vi "System_2.vi"() -> ()   [LabVIEW 2020]
doc: "Use this template to build a producer/consumer design pattern with events to produce queue items. Use this design pattern instead of the User Interface Event Handler pattern for user interfaces when you want to execute code asynchronously in response to an event without slowing the user interface responsiveness."
uses:
  <vilib>/Instr/_visa.llb/VISA Configure Serial Port (Instr).vi
panel:
  out "read data":string
  in  "Low LDR":dbl(slide) scale=0.0..1023.0
  in  "High LDR":dbl(slide) scale=0.0..1023.0
  out "Reward Servo":i32(knob) scale=0.0..180.0
  out "Forward Servo":i32(knob) scale=0.0..180.0
  in  "Baud rate (9600)":u32=9600
  in  "VISA resource name":refnum<visa-resource-name>
  in  "Close":bool
  in  "Open":bool
  out "Connected":bool
  in  "stop":bool
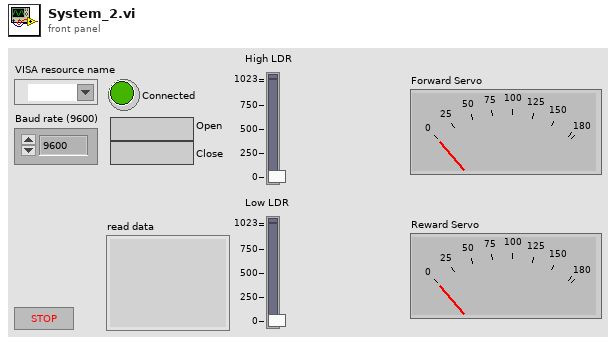
[diagram p1: front panel]
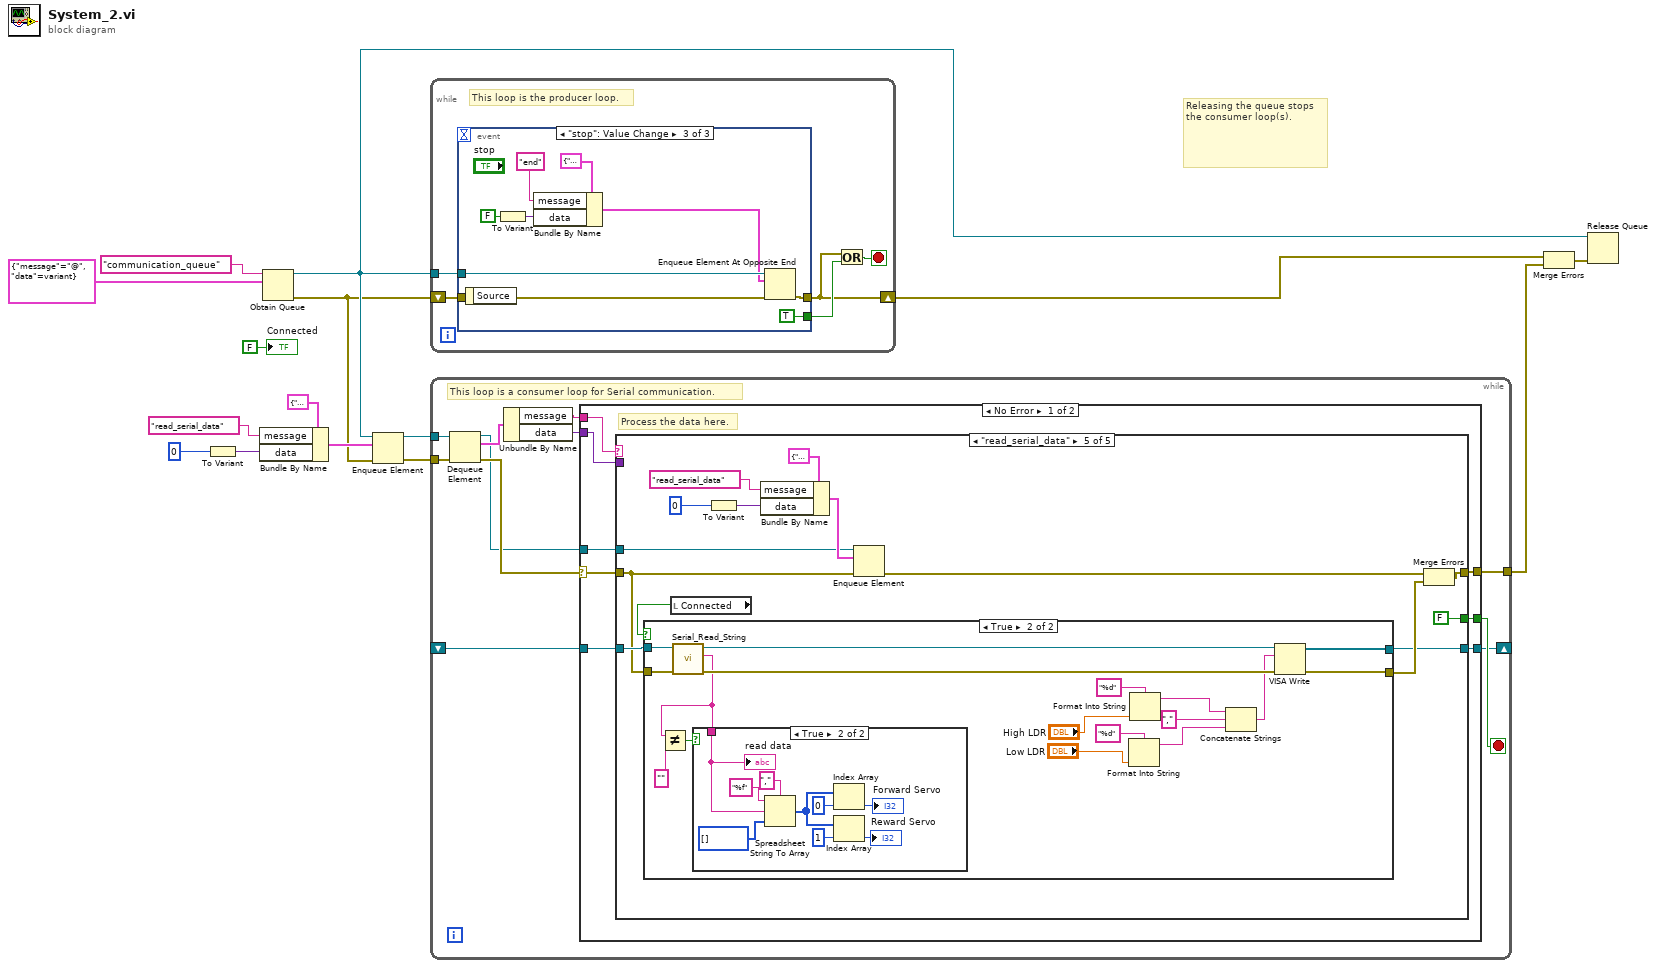
[diagram p0: block diagram]
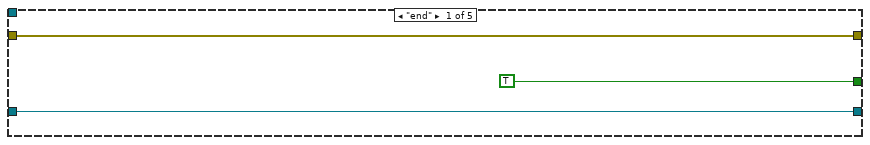
[diagram p2: hidden frame]
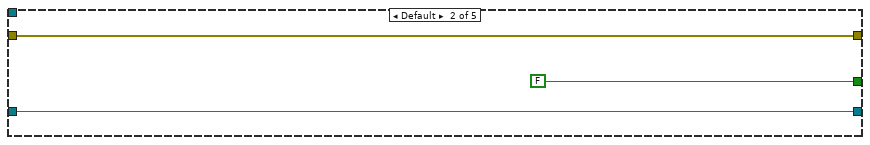
[diagram p3: hidden frame]
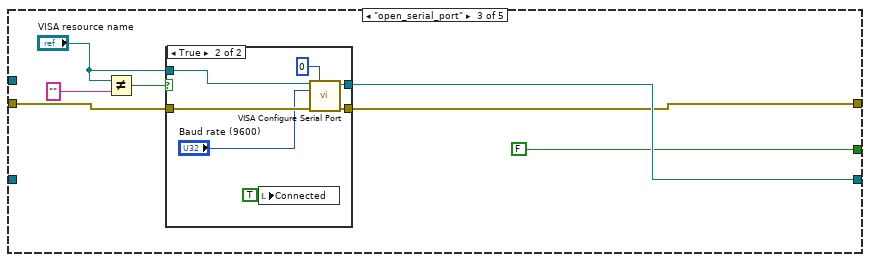
[diagram p4: hidden frame]
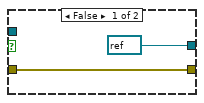
[diagram p5: hidden frame]
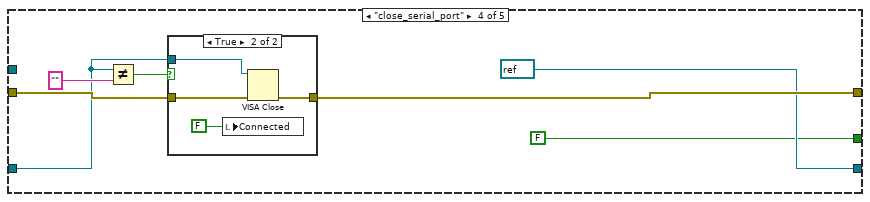
[diagram p6: hidden frame]
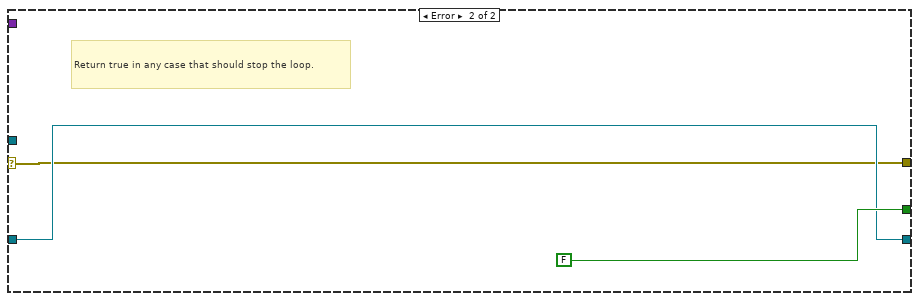
[diagram p10: hidden frame]
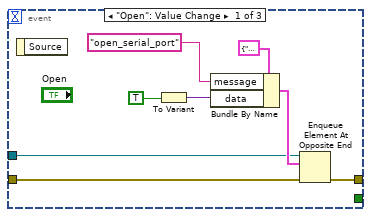
[diagram p11: hidden frame]
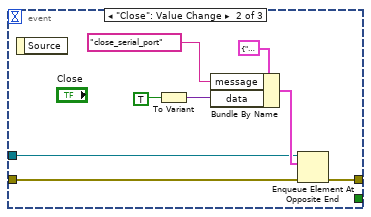
[diagram p12: hidden frame]
diagram:
  # "Releasing the queue stops the consumer loop(s)."
  n1 = To Variant(anything=0) -> (Variant=w8:variant)
  n2 = Bundle By Name(cluster=cluster{"message":string, "data":variant} {"message"="@", "data"=variant}, "message"="read_serial_data", "data"=w8) -> (w11:cluster{"message":string, "data":variant})
  n3 = Obtain Queue(name (unnamed)="communication_queue", element data type=cluster{"message":string, "data":variant} {"message"="@", "data"=variant}) -> (queue out=w4:refnum<queue>, error out=w1:errorcluster)  [unwired: 3 in, 1 out]
  n4 = Enqueue Element(queue=w4, element=w11, error in (no error)=w1) -> (queue out=w5:refnum<queue>, error out=w6:errorcluster)  [unwired: 1 in, 1 out]
  n5 = while {
    shift-right: [w17] -> w12
    shift-left: w1 -> [w20]
    tunnel: w4 -> [w16]
    stop <- w18 stop-if-true
    # "This loop is the producer loop."
    n6 = event shown="[2] \"stop\": Value Change" {
      selector: _ -> [_ _ _]
      dyn-events: _ -> [_ _ _]
      timeout: _ -> [_ _ _]
      tunnel: w20 -> [w24 w32 w38]
      tunnel: [w23 w31 w43] -> w17
      tunnel: [_ _ TRUE ("stop")] -> w19
      tunnel: w16 -> [w22 w30 w42]
      event "Open": Value Change {
        n7 = event-data() -> ()  [unwired: 1 in, 1 out]
        n8 = To Variant(anything=TRUE ("Open")) -> (Variant=w25:variant)
        n9 = Bundle By Name(cluster=cluster{"message":string, "data":variant} {"message"="@", "data"=variant}, "message"="open_serial_port", "data"=w25) -> (w28:cluster{"message":string, "data":variant})
        n10 = Enqueue Element At Opposite End(queue=w22, element=w28, error in (no error)=w24) -> (error out=w23:errorcluster)  [unwired: 1 in, 2 out]
      }
      event "Close": Value Change {
        n11 = event-data() -> ()  [unwired: 1 in, 1 out]
        n12 = To Variant(anything=TRUE ("Close")) -> (Variant=w33:variant)
        n13 = Bundle By Name(cluster=cluster{"message":string, "data":variant} {"message"="@", "data"=variant}, "message"="close_serial_port", "data"=w33) -> (w36:cluster{"message":string, "data":variant})
        n14 = Enqueue Element At Opposite End(queue=w30, element=w36, error in (no error)=w32) -> (error out=w31:errorcluster)  [unwired: 1 in, 2 out]
      }
      event "stop": Value Change {
        n15 = event-data() -> ()  [unwired: 1 in, 1 out]
        n16 = To Variant(anything=FALSE ("stop")) -> (Variant=w44:variant)
        n17 = Bundle By Name(cluster=cluster{"message":string, "data":variant} {"message"="@", "data"=variant}, "message"="end", "data"=w44) -> (w40:cluster{"message":string, "data":variant})
        n18 = Enqueue Element At Opposite End(queue=w42, element=w40, error in (no error)=w38) -> (error out=w43:errorcluster)  [unwired: 1 in, 2 out]
      }
    }
    n19 = Or(x=w17, y=w19) -> (x .or. y?=w18:bool)
  }
  n20 = while {
    tunnel: w5 -> [w56]
    tunnel: w6 -> [w52]
    shift-right: [w49] -> _
    shift-left: _ -> [w48]
    tunnel: [w47] -> w3
    stop <- w54 stop-if-true
    # "This loop is a consumer loop for Serial communication."
    n21 = Dequeue Element(queue=w56, error in (no error)=w52) -> (queue out=w46:refnum<queue>, element=w53:cluster{"message":string, "data":variant}, error out=w55:errorcluster)  [unwired: 1 in, 1 out]
    n22 = Unbundle By Name(w53) -> ("message"=w51:string, "data"=w50:variant)
    n23 = case shown="No Error" w55 {
      selector: w55 -> [w62 w141]
      tunnel: [w57 FALSE] -> w54
      tunnel: w51 -> [w64 _]
      tunnel: w50 -> [w63 _]
      tunnel: [w61 w142] -> w49
      tunnel: w48 -> [w60 w142]
      tunnel: [w59 w141] -> w47
      tunnel: w46 -> [w58 _]
      frame No Error {
        # "Process the data here."
        n24 = case shown="\"read_serial_data\"" w64 {
          tunnel: w63 -> [_ _ _ _ _]
          tunnel: w62 -> [w66 w69 w77 w93 w105]
          tunnel: [w67 w70 w73 refnum<visa-resource-name> refnum ("VISA resource name out") w100] -> w61
          tunnel: w60 -> [w67 w70 _ w90 w106]
          tunnel: [w66 w69 w72 w89 w103] -> w59
          tunnel: w58 -> [_ _ _ _ w108]
          tunnel: [TRUE FALSE FALSE FALSE FALSE] -> w57
          frame "end" {
          }
          frame Default {
          }
          frame "open_serial_port" {
            n25 = Not Equal?(x="VISA resource name", y="") -> (x != y?=w75:bool)
            n26 = case shown="True" w75 {
              tunnel: w77 -> [w78 w85]
              tunnel: "VISA resource name" -> [_ w82]
              tunnel: [refnum<visa-resource-name> refnum ("VISA resource name") w83] -> w73
              tunnel: [w78 w84] -> w72
              frame False {
              }
              frame True {
                n27 = local write "Connected"(TRUE ("Boolean")) -> ()
                n28 = call-poly "VISA Configure Serial Port"("VISA resource name"=w82, "timeout (10sec)"=u32 0, "baud rate (9600)"="Baud rate (9600)", "error in (no error)"=w85) -> ("VISA resource name out"=w83:refnum<visa-resource-name>, "error out"=w84:errorcluster)  [unwired: 10 in]
              }
            }
          }
          frame "close_serial_port" {
            n29 = Not Equal?(x=w90, y="") -> (x != y?=w91:bool)
            n30 = case shown="True" w91 {
              tunnel: w93 -> [w94 w98]
              tunnel: w90 -> [_ w97]
              tunnel: [w94 w95] -> w89
              frame False {
              }
              frame True {
                n31 = local write "Connected"(FALSE ("Boolean")) -> ()
                n32 = VISA Close(VISA resource name=w97, error in (no error)=w98) -> (error out=w95:errorcluster)
              }
            }
          }
          frame "read_serial_data" {
            n33 = local read "Connected"() -> (w99:bool)
            n34 = case shown="True" w99 {
              tunnel: w106 -> [w114 w131]
              tunnel: w105 -> [w113 w130]
              tunnel: [w113 w118] -> w101
              tunnel: [w114 w119] -> w100
              frame False {
              }
              frame True {
                n35 = call "Serial_Read_String.vi"("error in (no error)"=w130, "VISA Refnum in"=w131) -> ("error out"=w122:errorcluster, "read buffer"=w116:string, "VISA Refnum out"=w120:refnum<visa-resource-name>)  [unwired: 7 in]
                n36 = Not Equal?(x=w116, y="") -> (x != y?=w117:bool)
                n37 = case shown="True" w117 {
                  tunnel: w116 -> [_ w138]
                  frame False {
                  }
                  frame True {
                    n38 = Spreadsheet String To Array(delimiter (Tab)=",", format string="%f", spreadsheet string=w138, array type (2D Dbl)=i32[] [] ("default (0 I32)")) -> (array=w135:i32[])
                    n39 = Index Array(array=w135, index=0) -> (element=→"Forward Servo":i32)
                    n40 = Index Array(array=w135, index=1) -> (element=→"Reward Servo":i32)
                    "read data" <- w138
                  }
                }
                n41 = Format Into String(format string="%d", "Low LDR") -> (resulting string=w129:string)  [unwired: 2 in, 1 out]
                n42 = Format Into String(format string="%d", "High LDR") -> (resulting string=w128:string)  [unwired: 2 in, 1 out]
                n43 = Concatenate Strings(w128, "," ("string"), w129) -> (w121:string)
                n44 = VISA Write(VISA resource name=w120, write buffer=w121, error in (no error)=w122) -> (VISA resource name out=w119:refnum<visa-resource-name>, error out=w118:errorcluster)  [unwired: 1 out]
              }
            }
            n45 = To Variant(anything=0) -> (Variant=w109:variant)
            n46 = Bundle By Name(cluster=cluster{"message":string, "data":variant} {"message"="@", "data"=variant}, "message"="read_serial_data", "data"=w109) -> (w112:cluster{"message":string, "data":variant})
            n47 = Enqueue Element(queue=w108, element=w112, error in (no error)=w105) -> (error out=w104:errorcluster)  [unwired: 1 in, 2 out]
            n48 = Merge Errors(w104, w101) -> (w103:errorcluster)
          }
        }
      }
      frame Error {
        # "Return true in any case that should stop the loop."
      }
    }
  }
  n49 = Merge Errors(w12, w3) -> (w2:errorcluster)
  n50 = Release Queue(queue=w4, error in (no error)=w2) -> ()  [unwired: 1 in, 3 out]
  "Connected" <- FALSE ("Boolean")
